vi "EndService.vi"(1 "In":i32) -> (0 "Out":i32)   [LabVIEW 2011]
doc: "Copyright (c) 2005, Kuan Chen\nAll rights reserved.\n\nRedistribution and use in source and binary forms, with or without modification, are permitted provided that the following conditions are met:\n\n * Redistributions of source code must retain the above copyright notice, this list of conditions and the following disclaimer.\n * Redistributions in binary form must reproduce the above copyright notice, this list of conditions and the following disclaimer in the documentation and/or other materials provided with the distribution.\n * Neither the name of the Kuan Chen nor the names of its contributors may be used to endorse or promote products derived from this software without specific prior written permission.\n\nTHIS SOFTWARE IS PROVIDED BY THE COPYRIGHT HOLDERS AND CONTRIBUTORS \"AS IS\" AND ANY EXPRESS OR IMPLIED WARRANTIES, INCLUDING, BUT NOT LIMITED TO, THE IMPLIED WARRANTIES OF MERCHANTABILITY AND FITNESS FOR A PARTICULAR PURPOSE ARE DISCLAIMED. IN NO EVENT SHALL THE COPYRIGHT OWNER OR CONTRIBUTORS BE LIABLE FOR ANY DIRECT, INDIRECT, INCIDENTAL, SPECIAL, EXEMPLARY, OR CONSEQUENTIAL DAMAGES (INCLUDING, BUT NOT LIMITED TO, PROCUREMENT OF SUBSTITUTE GOODS OR SERVICES; LOSS OF USE, DATA, OR PROFITS; OR BUSINESS INTERRUPTION) HOWEVER CAUSED AND ON ANY THEORY OF LIABILITY, WHETHER IN CONTRACT, STRICT LIABILITY, OR TORT (INCLUDING NEGLIGENCE OR OTHERWISE) ARISING IN ANY WAY OUT OF THE USE OF THIS SOFTWARE, EVEN IF ADVISED OF THE POSSIBILITY OF SUCH DAMAGE.\n\nStops the OutputThread.vi from continuing to output to the output file. Returns 0."
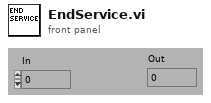
[diagram p1: front panel]
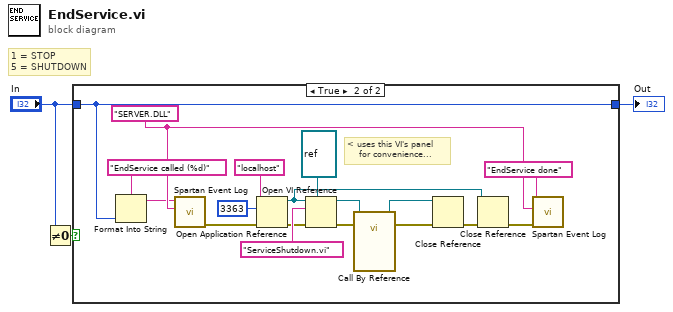
[diagram p0: block diagram]
diagram:
  # "1 = STOP\n5 = SHUTDOWN"
  n1 = Not Equal To 0?(x="In") -> (x != 0?=w3:bool)
  n2 = case shown="True" w3 {
    tunnel: "In" -> [w4 w18]
    tunnel: [w4 w18] -> w1
    frame False {
    }
    frame True {
      w22 = "SERVER.DLL" ("message (\"\")")
      # "< uses this VI's panel\n    for convenience..."
      n3 = Format Into String(format string="EndService called (%d)" ("message (\"\")"), w18) -> (resulting string=w19:string)  [unwired: 2 in, 1 out]
      n4 = call "Spartan Event Log.vi"("module (\"\")"=w22, "message (\"\")"=w19) -> ("error out"=w14:errorcluster)  [unwired: 3 in, 3 out]
      n5 = Open Application Reference(8:w14, 10:u16 3363 ("port number or service name (3363)"), 11:"localhost" ("message (\"\")")) -> (0:w13:errorcluster, 3:w6:refnum<vi>)  [unwired: 1 in]
      n6 = Open VI Reference(type specifier VI Refnum (for type only)=refnum<vi> refnum, application reference (local)=w6, vi path="ServiceShutdown.vi" ("message (\"\")"), error in (no error)=w13) -> (vi reference=w9:refnum<vi>, error out=w7:errorcluster)  [unwired: 2 in]
      n7 = call-by-ref "?"(reference=w9, error in=w7) -> (reference out=w8:refnum<vi>, error out=w15:errorcluster)  [unwired: 1 in, 1 out]
      n8 = Close Reference(reference=w8, error in (no error)=w15) -> (error out=w5:errorcluster)
      n9 = Close Reference(reference=w6, error in (no error)=w5) -> (error out=w12:errorcluster)
      n10 = call "Spartan Event Log.vi"("error in (no error)"=w12, "module (\"\")"=w22, "message (\"\")"="EndService done" ("message (\"\")")) -> ()  [unwired: 2 in, 4 out]
    }
  }
  "Out" <- w1
